vi "FiberSpectrograph_putSample_exists.vi"(8 "error in (no error)":errorcluster, 11 "exists_Ctl":T1) -> (0 "error out":errorcluster, 2 "function return":i32, 3 "exists_Ctl out":T1)   [LabVIEW 2016, in "SALLV_FiberSpectrograph.lvlib"]
doc: "int FiberSpectrograph_shm_putSample_existsLV(FiberSpectrograph_existsLV *exists_Ctl );"
uses:
  SALLV_FiberSpectrograph.lvlib
  DataTypes/exists.ctl
  SALLV_FiberSpectrograph.so
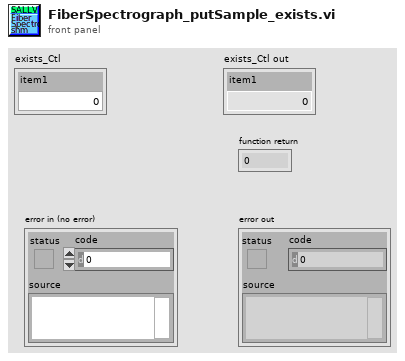
[diagram p1: front panel]
types:
  T1 = typedef "SALLV_FiberSpectrograph.lvlib/exists.ctl" = cluster{"item1":i32}
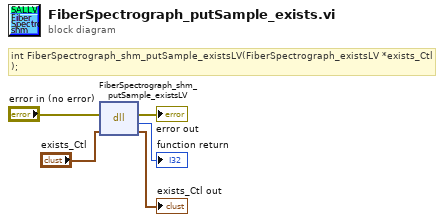
[diagram p0: block diagram]
diagram:
  # "int FiberSpectrograph_shm_putSample_existsLV(FiberSpectrograph_existsLV *exists_Ctl );"
  n1 = dll-call lib="home/harini/Documents/lsst/SALLV_FiberSpectrograph/SALLV_FiberSpectrograph.*" fn="FiberSpectrograph_shm_putSample_existsLV"(error in="error in (no error)", "exists_Ctl"="exists_Ctl") -> (error out=→"error out":errorcluster, →"function return":i32, "exists_Ctl"=→"exists_Ctl out":T1)  [unwired: 2 in, 1 out]
